vi "simulate_osc.vi"(7 "CHAN":T2={"channel name"="CHANNEL2", "probe attenuation"=1.0, "vertical offset"=0.0, "vertical range"=1.0, "vertical coupling"=1, "input impedance"=50.0} {"input impedance" format="%#_13g"; "vertical coupling" items=["AC", "DC", "GND"]; "vertical range" format="%.3f"; "vertical offset" format="%.3f"; "probe attenuation" format="%.3f"}, 10 "trace":T1={"N"=700, "x0"=-1e-07, "dx"=9.999999999999999e-10, "noise"=0.002, "A"=1.0, "eff"=0.25, "sigma"=10.0, "tau"=142.0} {"dx" format="%#_13g"; "noise" format="%#_13g"}) -> (2 "output waveform":waveform(dbl)={"t0"=timestamp(0 s since 1904-01-01), "dt"=1e-08, "Y"=array[1000 elements]})   [LabVIEW 2015, in "oscilloscope.lvlib"]
uses:
  oscilloscope.lvlib
  osc_channel.ctl
  simulate_trace.ctl
panel:
  out "min":dbl=-0.5
  out "max":dbl=0.5
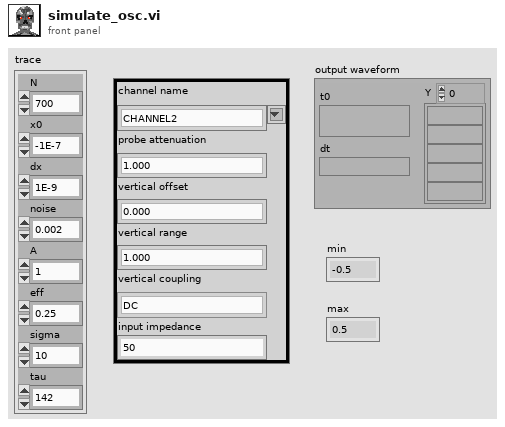
[diagram p1: front panel]
types:
  T1 = typedef "oscilloscope.lvlib/simulate_trace.ctl" = cluster{"N":i32, "x0":dbl, "dx":dbl, "noise":dbl, "A":dbl, "eff":dbl, "sigma":dbl, "tau":dbl}
  T2 = typedef "oscilloscope.lvlib/osc_channel.ctl" = cluster{"channel name":string, "probe attenuation":dbl, "vertical offset":dbl, "vertical range":dbl, "vertical coupling":i32, "input impedance":dbl}
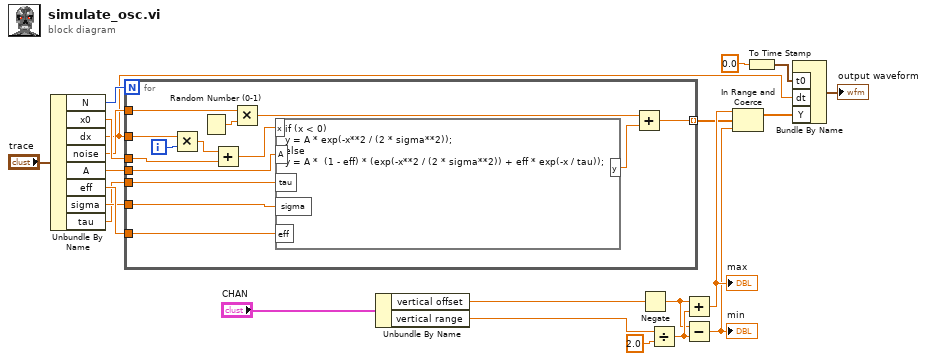
[diagram p0: block diagram]
diagram:
  n1 = Unbundle By Name("trace") -> ("N"=w8:i32, "x0"=w7:dbl, "dx"=w1:dbl, "noise"=w6:dbl, "A"=w5:dbl, "eff"=w4:dbl, "sigma"=w3:dbl, "tau"=w2:dbl)
  n2 = for {
    N: w8 -> [_]
    tunnel: [w30] -> w10 mode=indexing
    tunnel: w7 -> [w29]
    tunnel: w1 -> [w28]
    tunnel: w6 -> [w27]
    tunnel: w5 -> [w26]
    tunnel: w4 -> [w25]
    tunnel: w3 -> [w24]
    tunnel: w2 -> [w23]
    i -> [w36]
    n3 = Multiply(x=w28, y=w36) -> (x*y=w35:dbl)
    n4 = Random Number (0-1)() -> (number: 0 to 1=w32:dbl)
    n5 = Add(x=w35, y=w29) -> (x+y=w34:dbl)
    n6 = Multiply(x=w27, y=w32) -> (x*y=w33:dbl)
    n7 = formula code="if (x < 0)\ny = A * exp(-x**2 / (2 * sigma**2));\nelse\ny = A *  (1 - eff) * (exp(-x**2 / (2 * sigma**2)) + eff * exp(-x / tau));"("x"=w34, "tau"=w23, "sigma"=w24, "eff"=w25, "A"=w26) -> ("y"=w31:dbl)
    n8 = Add(x=w33, y=w31) -> (x+y=w30:dbl)
  }
  n9 = Unbundle By Name("CHAN") -> ("vertical offset"=w15:dbl, "vertical range"=w18:dbl)
  n10 = Negate(x=w15) -> (-x=w14:dbl)
  n11 = Divide(x=w18, y=2.0) -> (x/y=w16:dbl)
  n12 = Add(x=w14, y=w16) -> (x+y=w13:dbl)
  "max" <- w13
  n13 = Subtract(x=w14, y=w16) -> (x-y=w12:dbl)
  "min" <- w12
  n14 = In Range and Coerce(upper limit=w13, x=w10, lower limit=w12) -> (coerced(x)=w20:dbl[])  [unwired: 1 out]
  n15 = To Time Stamp(1:0.0 ("number")) -> (0:w22:timestamp)
  n16 = Bundle By Name("t0"=w22, "dt"=w1, "Y"=w20) -> (→"output waveform":waveform(dbl))  [unwired: 1 in]
